vi "rszvl Query Marker.vi"(8 "error in (no error)":errorcluster, 9 "Marker (1)":i32=1, 10 "Channel (1)":i32=1, 11 "VISA resource name":refnum<visa-resource-name>) -> (0 "error out":errorcluster, 1 "Marker Amplitude":dbl format="%^.3e", 2 "Marker Position":dbl format="%^.3e", 3 "VISA resource name out":refnum<visa-resource-name>)   [LabVIEW 2014]
doc: "This VI returns the horizontal position and the marker amplitude level of the selected marker.\n\nAttribute(s):\nRSZVL_ATTR_NWA_MARKER_POSITION\nRSZVL_ATTR_NWA_MARKER_AMPLITUDE\n\nRemote-control command(s):\nCALCulate<Chn>:MARKer<Mk>:X?\nCALCulate<Chn>:MARKer<Mk>:Y?"
uses:
  Instance           2 26Saved   rszvl Query Marker .vi
  Instance           3 26Saved   rszvl Query Marker .vi
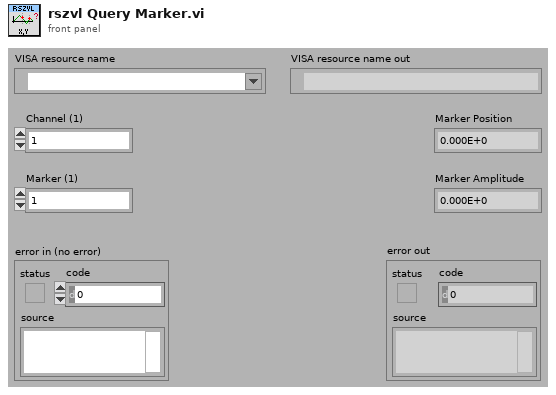
[diagram p1: front panel]
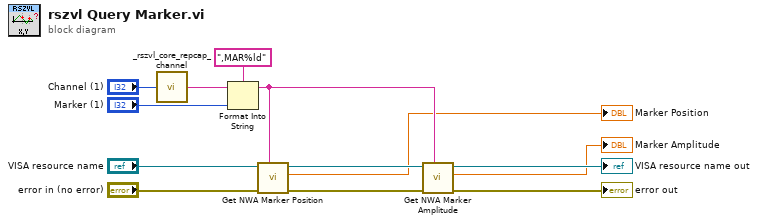
[diagram p0: block diagram]
diagram:
  n1 = call "_rszvl_core_repcap_channel.vi"("Channel"="Channel (1)") -> ("Rep cap"=w12:string)
  n2 = Format Into String(format string=",MAR%ld", initial string=w12, "Marker (1)") -> (resulting string=w5:string)  [unwired: 1 in, 1 out]
  n3 = call "Get NWA Marker Position"("Repeated Capabilities"=w5, "error in (no error)"="error in (no error)", "instrument handle"="VISA resource name") -> ("error out"=w6:errorcluster, "NWA Marker Position"=→"Marker Position":dbl, "instrument handle out"=w7:refnum<visa-resource-name>)  [unwired: 6 in]
  n4 = call "Get NWA Marker Amplitude"("Repeated Capabilities"=w5, "error in (no error)"=w6, "instrument handle"=w7) -> ("error out"=→"error out":errorcluster, "NWA Marker Amplitude"=→"Marker Amplitude":dbl, "instrument handle out"=→"VISA resource name out":refnum<visa-resource-name>)  [unwired: 6 in]
